vi "Queueu Comms Enqueue.vi"(8 "error in":errorcluster, 11 "Element":T1={"Estados"=enum."inicio", "Data"=variant}) -> (0 "error out":errorcluster, 3 "queue out":refnum<queue>)   [LabVIEW 2019]
doc: "Este VI pone elementos en la cola."
uses:
  Private Controls/Control HMI Data Cluster.ctl
  Private Controls/Estados.ctl
  Private Controls/Queue FGV Action.ctl
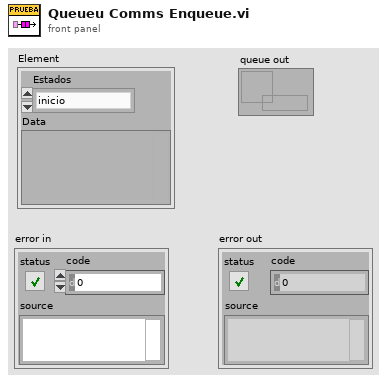
[diagram p1: front panel]
types:
  T1 = typedef "Control HMI Data Cluster.ctl" = cluster{"Estados":T2, "Data":variant}
  T2 = typedef "Estados.ctl" = enum16{"CargaReferencias", "LeerArchivoConfiguracion", "RevisaTipoGenerador", "inicio", "conf_instru", "escribe_frec", "lee_BD", "lee_referencia", "guardarVrefA", "guardarVrefC", "guardarVrefZ", "FrecAmp_A1", "FrecAmp_C1", "FrecAmp_Z1", "FrecAmp_A2", "FrecAmp_C2", "FrecAmp_Z2", "iniciarGEN", "monitoreo", "detenerGEN", "crea_voltajes_prueba_A", "crea_voltajes_prueba_C", "crea_voltajes_prueba_Z", "voltajeInicialA2", "voltajeInicialC2", "voltajeInicialZ2", "actualizarVrefA", "actualizarVrefC", "actualizarVrefZ", "ingresaMedicionesA", "ingresaMedicionesC", "ingresaMedicionesZ", "cumplimiento", "listo_evaluar", "evaluar", "final", "guardaMedicionesA", "guardaMedicionesC", "guardaMedicionesZ", "ultimaFrec", "generaA2", "detieneA2", "salir", "Error"}
  T3 = typedef "Queue FGV Action.ctl" = enum16{"Set", "Get", "Release"}
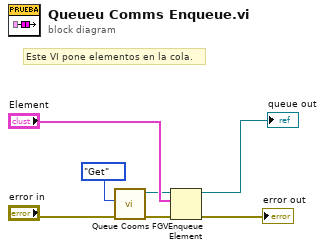
[diagram p0: block diagram]
diagram:
  # "Este VI pone elementos en la cola."
  n1 = call "Queue Cooms FGV.vi"("error in"="error in", "Action"=Queue_FGV_Action."Get") -> ("error out"=w6:errorcluster, "queue out"=w5:refnum<queue>)  [unwired: 8 in]
  n2 = Enqueue Element(queue=w5, element="Element", error in (no error)=w6) -> (queue out=→"queue out":refnum<queue>, error out=→"error out":errorcluster)  [unwired: 1 in, 1 out]
